vi "from string.vi"(8 "error in":errorcluster, 9 "data":string, 10 "version":string, 11 "OPC UA configuration in":refnum<class "OPC UA Server configuration.lvclass">) -> (0 "error out":errorcluster, 3 "OPC UA configuration out":refnum<class "OPC UA Server configuration.lvclass">)   [LabVIEW 2013, in "OPC UA Server configuration.lvclass"]
doc: "Provides an interface for loading a module configuration from a file or other serialized data source. It is recommended that all children of this class store data in two sets--data required for its own initialization, and any data required for parent initialization--and that each implementation uses the <b>Call Parent Method</b> primitive to de-serialize parent information. As a result, it is expected that every module configuration class calls <b>component configuration.lvclass:From String.vi</b>."
uses:
  OPC UA Server configuration.lvclass
  Line.ctl
  <vilib>/NI/Tag Bus Module Framework/channel/TBM channel.lvclass
  OPC UA Data Type.ctl
  <vilib>/OPCUA/server/subVI/supported security policies.ctl
  <vilib>/NI/Tag Bus Module Framework/module configuration/TBM module configuration.lvclass
  OPC UA Server configuration.lvclass/OPC UA Server configuration.ctl
  <vilib>/NI/Configuration Framework/serializable configuration/NISE_CEF_serializable configuration.lvclass
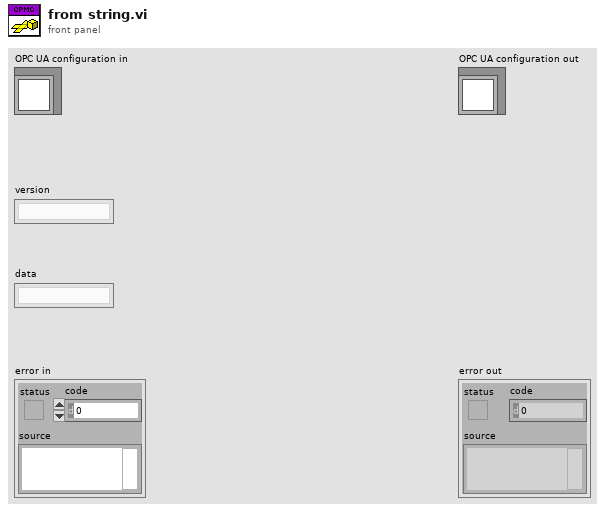
[diagram p1: front panel]
types:
  T1 = typedef "OPC UA Server configuration.lvclass/Line.ctl" = cluster{"channel":refnum<class "TBM channel.lvclass">, "Node Path":string, "OPC UA Data Type":T2}
  T2 = typedef "OPC UA Server configuration.lvclass/OPC UA Data Type.ctl" = u16
  T3 = typedef "supported security policies.ctl" = cluster{"None":bool, "Sign with Basic128Rsa125":bool, "Sign and Encrypt with Basic128Rsa125":bool, "Sign with Basic256":bool, "Sign and Encrypt with Basic256":bool}
  T4 = cluster{"Client?":bool, "Server Certificates":cluster{"Relative Path?":bool, "Certificate Paths":path[], "Certificate Names":string[]}, "Client Certificates":cluster{"Relative Path?":bool, "Certificate Paths":path[], "Certificate Names":string[]}, "Client Configuration":cluster{"Server Endpoint URL":string, "Security Policy":cluster{"Message Mode":enum16{"None", "Sign", "Sign and Encrypt"}, "Security":enum16{"Basic256", "Basic128Rsa15"}}, "Username/Password":cluster{"Username":string, "Password":string}}, "Server Configuration":cluster{"Server Name":string, "TCP port (49580)":string, "Supported Security Policies":T3}}
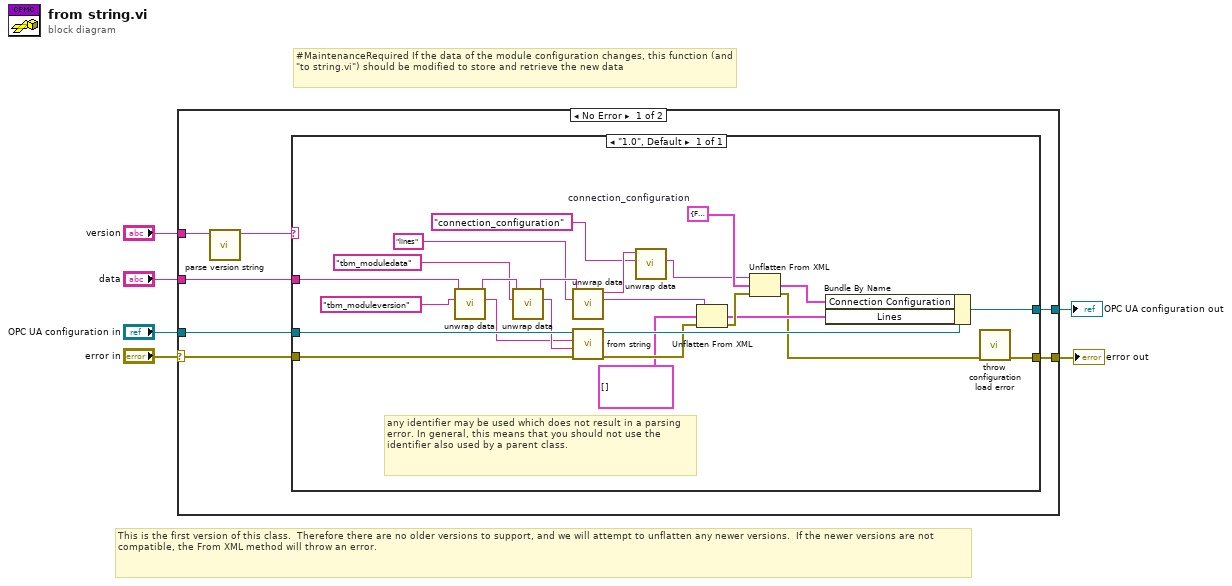
[diagram p0: block diagram]
diagram:
  # "#MaintenanceRequired If the data of the module configuration changes, this function (and \"to string.vi\") should be modified to store and retrieve the new data"
  # "This is the first version of this class.  Therefore there are no older versions to support, and we will attempt to unflatten any newer versions.  If the newer versions are not compatible, the From XML method will throw an error."
  n1 = case shown="No Error" "error in" {
    selector: "error in" -> [w7 w39]
    tunnel: "data" -> [w13 _]
    tunnel: "OPC UA configuration in" -> [w12 w38]
    tunnel: [w11 w38] -> w5
    tunnel: [w10 w39] -> w4
    tunnel: "version" -> [w9 _]
    frame No Error {
      n2 = call <vilib>:"parse version string.vi"("full version"=w9) -> ("major.minor version"=w8:string)  [unwired: 7 in, 3 out]
      n3 = case shown="\"1.0\", Default" w8 {
        tunnel: w13 -> [w34]
        tunnel: w7 -> [w33]
        tunnel: w12 -> [w37]
        tunnel: [w25] -> w11
        tunnel: [w36] -> w10
        frame "1.0", Default {
          w17 = T4 {"Client?"=FALSE, "Server Certificates"={"Relative Path?"=FALSE, "Certificate Paths"=[], "Certificate Names"=[]}, "Client Certificates"={"Relative Path?"=FALSE, "Certificate Paths"=[], "Certificate Names"=[]}, "Client Configuration"={"Server Endpoint URL"="", "Security Policy"={"Message Mode"=enum."None", "Security"=enum."Basic256"}, "Username/Password"={"Username"="", "Password"=""}}, "Server Configuration"={"Server Name"="", "TCP port (49580)"="", "Supported Security Policies"={"None"=FALSE, "Sign with Basic128Rsa125"=FALSE, "Sign and Encrypt with Basic128Rsa125"=FALSE, "Sign with Basic256"=FALSE, "Sign and Encrypt with Basic256"=FALSE}}}  # connection_configuration
          # "any identifier may be used which does not result in a parsing error. In general, this means that you should not use the identifier also used by a parent class."
          n4 = call <vilib>:"unwrap data.vi"("identifier"="tbm_moduleversion" ("additional identifier"), "data to unwrap"=w34) -> ("unwrapped data"=w29:string, "remaining string"=w35:string)  [unwired: 8 in]
          n5 = call <vilib>:"unwrap data.vi"("identifier"="tbm_moduledata" ("additional identifier"), "data to unwrap"=w35) -> ("unwrapped data"=w31:string, "remaining string"=w28:string)  [unwired: 8 in]
          n6 = call <vilib>:"unwrap data.vi"("identifier"="lines" ("additional identifier"), "data to unwrap"=w28) -> ("unwrapped data"=w24:string, "remaining string"=w21:string)  [unwired: 8 in]
          n7 = call-parent "from string.vi"("error in"=w33, "data"=w31, "version"=w29, "module configuration in"=w37) -> ("error out"=w23:errorcluster, "module configuration out"=w26:refnum<class "OPC UA Server configuration.lvclass">)  [unwired: 6 in]
          n8 = call <vilib>:"unwrap data.vi"("identifier"="connection_configuration" ("additional identifier"), "data to unwrap"=w21) -> ("unwrapped data"=w14:string)  [unwired: 8 in, 1 out]
          n9 = Unflatten From XML(xml string=w24, type=T1[] [] ("Lines"), error in (no error)=w23) -> (value=w18:T1[], error out=w19:errorcluster)
          n10 = Unflatten From XML(xml string=w14, type=w17, error in (no error)=w19) -> (value=w15:T4, error out=w16:errorcluster)
          n11 = Bundle By Name(cluster=w26, "Connection Configuration"=w15, "Lines"=w18) -> (w25:refnum<class "OPC UA Server configuration.lvclass">)
          n12 = call <vilib>:"throw configuration load error.vi"("error in"=w16) -> ("error out"=w36:errorcluster)  [unwired: 10 in]
        }
      }
    }
    frame Error {
    }
  }
  "error out" <- w4
  "OPC UA configuration out" <- w5
